vi "FMA1600A Meter Present.vi"(5 "SLPM Error @ Zero":dbl, 7 "Unit ID":string, 8 "error in (no error)":errorcluster, 9 "Meter Present":bool, 11 "VISA Refnum in":refnum<visa-resource-name>) -> (0 "error out":errorcluster, 2 "FMA1600A Gas Data":T1)   [LabVIEW 2018]
uses:
  Type Definitions/FMA1600A Data.ctl
  Type Definitions/FMA1600A Commands.ctl
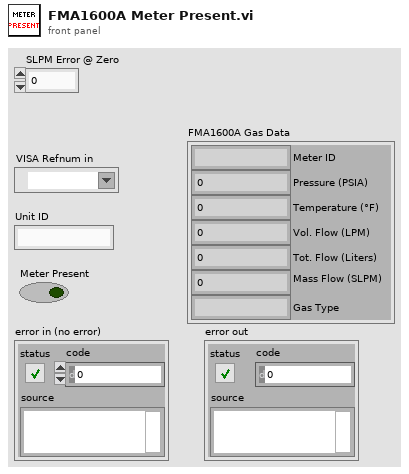
[diagram p1: front panel]
types:
  T1 = typedef "FMA1600A Data.ctl" = cluster{"Pressure (PSIA)":dbl, "Temperature (°F)":dbl, "Vol. Flow (LPM)":dbl, "Mass Flow (SLPM)":dbl, "Gas Type":string, "Tot. Flow (Liters)":dbl, "Meter ID":string}
  T2 = typedef "FMA1600A Commands.ctl" = string
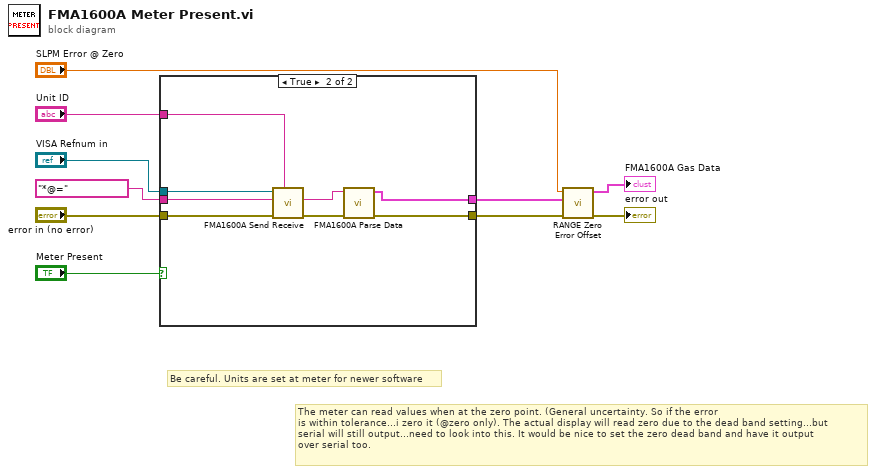
[diagram p0: block diagram]
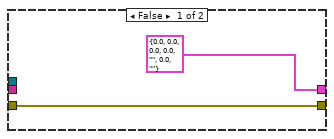
[diagram p2: hidden frame]
diagram:
  # "Be careful. Units are set at meter for newer software"
  # "The meter can read values when at the zero point. (General uncertainty. So if the error\nis within tolerance...i zero it (@zero only). The actual display will read zero due to the dead band setting...but\nserial will still output...need to look into this. It would be nice to set the zero dead band and have it output\nover serial too."
  n1 = case shown="True" "Meter Present" {
    tunnel: [T1 {"Pressure (PSIA)"=0.0, "Temperature (°F)"=0.0, "Vol. Flow (LPM)"=0.0, "Mass Flow (SLPM)"=0.0, "Gas Type"="", "Tot. Flow (Liters)"=0.0, "Meter ID"=""} ("FMA1600A Gas Data") w20] -> w5
    tunnel: T2 "*@=" ("FMA1600A Commands") -> [_ w19]
    tunnel: "error in (no error)" -> [w12 w18]
    tunnel: [w12 w13] -> w2
    tunnel: "VISA Refnum in" -> [_ w17]
    tunnel: "Unit ID" -> [_ w14]
    frame False {
    }
    frame True {
      n2 = call "FMA1600A Send Receive.vi"("Unit ID"=w14, "error in (no error)"=w18, "FMA1600A Commands"=w19, "VISA Refnum in"=w17) -> ("error out"=w16:errorcluster, "Raw FMA1600A Data"=w15:string)  [unwired: 5 in, 1 out]
      n3 = call "FMA1600A Parse Data.vi"("Error In"=w16, "Raw FMA1600A Data"=w15) -> ("Error Out"=w13:errorcluster, "FMA1600A Gas Data"=w20:T1)  [unwired: 7 in]
    }
  }
  n4 = call "RANGE Zero Error Offset.vi"("Error In"=w2, "FMA1600A Gas Data in"=w5, "SLPM Error @ Zero"="SLPM Error @ Zero") -> ("Error Out"=→"error out":errorcluster, "FMA1600A Gas Data out"=→"FMA1600A Gas Data":T1)  [unwired: 7 in]
